vi "CMC-InClass-Enhanced Square Root.vi"() -> ()   [LabVIEW 2010]
panel:
  out "Square Root":dbl
  in  "Input Value":dbl
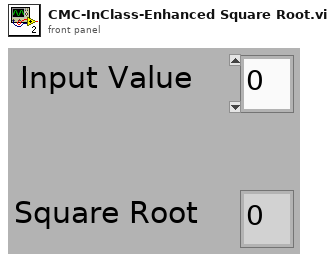
[diagram p1: front panel]
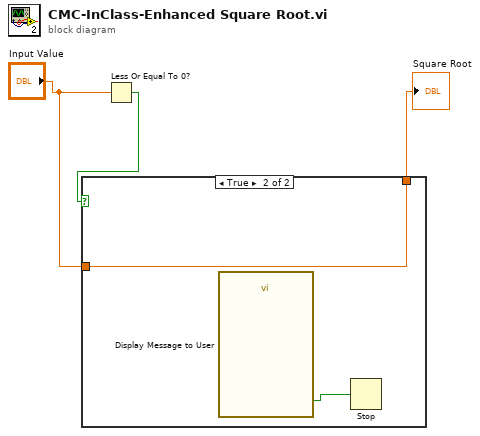
[diagram p0: block diagram]
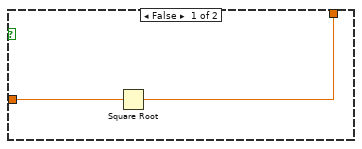
[diagram p2: hidden frame]
diagram:
  n1 = Less Or Equal To 0?(x="Input Value") -> (x <= 0?=w3:bool)
  n2 = case shown="True" w3 {
    tunnel: "Input Value" -> [w5 w7]
    tunnel: [w4 w7] -> w1
    frame False {
      n3 = Square Root(x=w5) -> (sqrt(x)=w4:dbl)
    }
    frame True {
      n4 = call "Display Message to User"() -> ("OK"=w6:bool)  [unwired: 10 in, 1 out]
      n5 = Stop(stop? (T)=w6) -> ()
    }
  }
  "Square Root" <- w1
